vi "Image_Filter_Red.vi"(0 "Input Image":T1, 1 "New Image of IMAQ Threshold":T1, 2 "New Image for Color Threshold":T1) -> (4 "Output Image of Object Detection":T1, 6 "Objects":T2(array[cluster]) {"Aspect Ratio" format="%.2f"; "Orientation" format="%.2f"; "Area" format="%.2f"; "Object Center"."Y" format="%.2f"; "Object Center"."X" format="%.2f"}, 7 "Number of Objects":i32)   [LabVIEW 2015]
uses:
  <vilib>/vision/Image Controls.llb/IMAQ Image.ctl
  <vilib>/vision/NI_Vision_Development_Module.lvlib
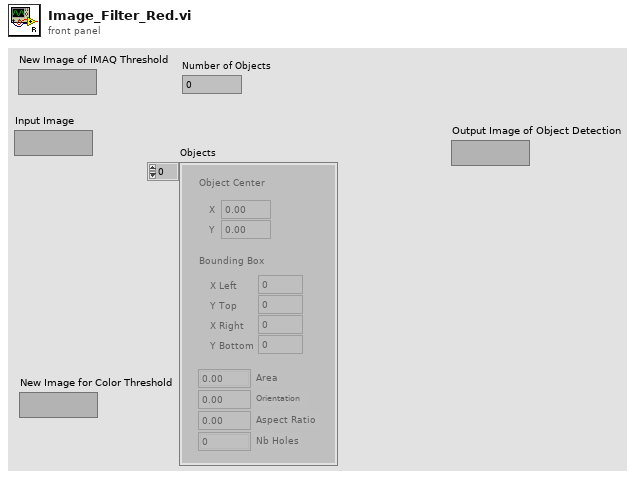
[diagram p1: front panel]
types:
  T1 = typedef "IMAQ Image.ctl" = refnum<image>
  T2 = cluster{"Object Center":cluster{"X":sgl, "Y":sgl}, "Bounding Box":cluster{"X Left":i32, "Y Top":i32, "X Right":i32, "Y Bottom":i32}, "Area":sgl, "Orientation":sgl, "Aspect Ratio":sgl, "Nb Holes":i32}[]
  T3 = cluster{"Objects":u16, "Threshold":i32, "Reject Border":bool, "Fill Holes":bool, "Min Object Size":bool, "Min Size":i32, "Max Object Size":bool, "Max Size":i32, "Show Search Area":bool, "Show Center":bool, "Show Bounding Box":bool}
  T4 = enum32{"AutoM", "Close", "Dilate", "Erode", "Gradient", "Gradient out", "Gradient in", "Hit miss", "Open", "PClose", "POpen", "Thick", "Thin"}
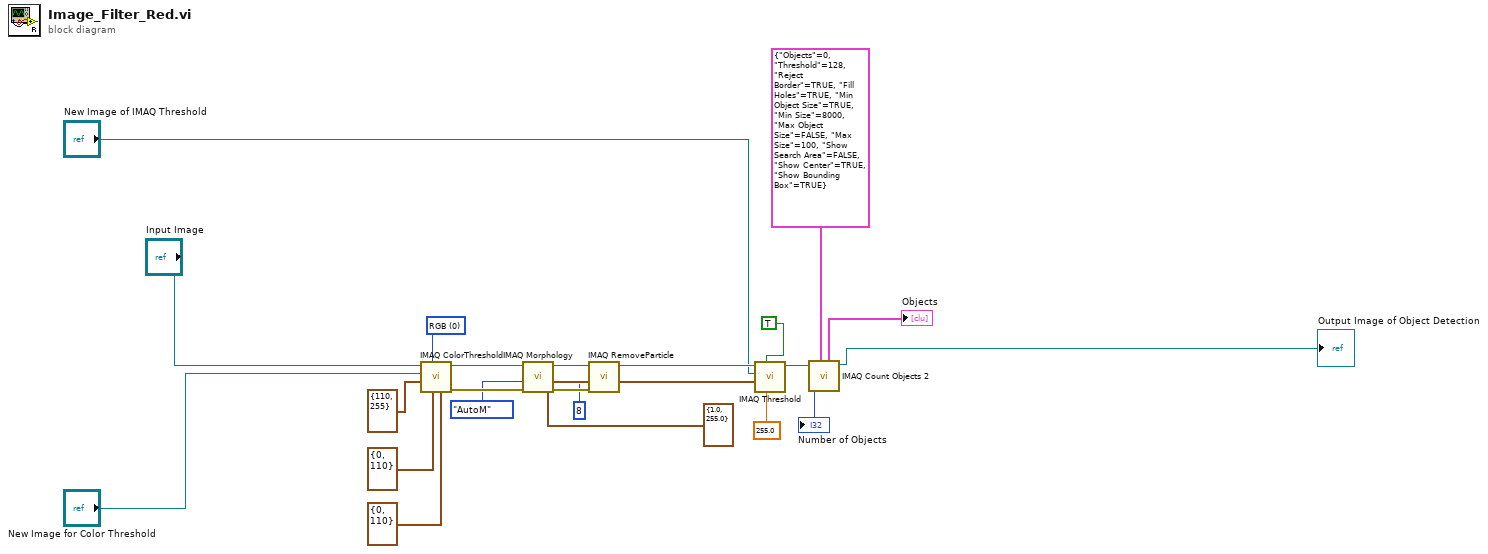
[diagram p0: block diagram]
diagram:
  w1 = u16 0 items=["RGB", "HSL", "HSV", "HSI"] ("Color Mode")
  n1 = call "IMAQ ColorThreshold"("Blue or Luma or Val or Inten Range"=cluster{"Lower value":i32, "Upper value":i32} {"Lower value"=0, "Upper value"=110}, "Green or Sat Range"=cluster{"Lower value":i32, "Upper value":i32} {"Lower value"=0, "Upper value"=110}, "Color Mode"=w1, "Red or Hue Range"=cluster{"Lower value":i32, "Upper value":i32} {"Lower value"=110, "Upper value"=255}, "Image Dst"="New Image for Color Threshold", "Image Src"="Input Image") -> ("error out"=w9:errorcluster, "Image Dst Out"=w11:T1)  [unwired: 4 in]
  n2 = call "IMAQ Morphology"("error in (no error)"=w9, "Operation"=T4."AutoM", "Image Src"=w11) -> ("error out"=w10:errorcluster, "Image Dst Out"=w7:T1)  [unwired: 4 in, 3 out]
  n3 = call "IMAQ RemoveParticle"("error in (no error)"=w10, "Number of Erosion"=8, "Image Src"=w7) -> ("Image Dst Out"=w16:T1)  [unwired: 4 in, 4 out]
  n4 = call "IMAQ Threshold"("Replace Value"=sgl 255.0, "Keep/Replace Value (Replace)"=TRUE, "Range"=cluster{"Lower value":sgl, "Upper value":sgl} {"Lower value"=1.0, "Upper value"=255.0}, "Image Dst"="New Image of IMAQ Threshold", "Image Src"=w16) -> ("Image Dst Out"=w20:T1)  [unwired: 5 in, 1 out]
  n5 = call "IMAQ Count Objects 2"("Settings"=T3 {"Objects"=0, "Threshold"=128, "Reject Border"=TRUE, "Fill Holes"=TRUE, "Min Object Size"=TRUE, "Min Size"=8000, "Max Object Size"=FALSE, "Max Size"=100, "Show Search Area"=FALSE, "Show Center"=TRUE, "Show Bounding Box"=TRUE}, "Image"=w20) -> ("Number of Objects"=→"Number of Objects":i32, "Image Out"=→"Output Image of Object Detection":T1, "Objects"=→"Objects":T2)  [unwired: 5 in, 2 out]
